vi "MdbPosEchoTableToCsv_topLevel.vi"() -> ()   [LabVIEW 2011]
uses:
  <vilib>/Utility/sysdir.llb/System Directory Type.ctl
  <vilib>/addons/database/Connection.llb/DB Tools Open Connec (String).vi
  <vilib>/addons/database/Connection.llb/DB Tools Open Connec (Path).vi
  <vilib>/addons/database/Connection.llb/Conn Get Properties.vi
  <vilib>/addons/database/_DB Variant To Data/Database Variant To Data.xnode
  <vilib>/addons/database/NI_Database_API.lvlib
panel:
  in  "Footer":string
  in  "Header":string
  in  "Database Setup":bool
  out "NumberLeft":i32 caption="Number Left To Process"
  in  "Run":bool
  in  "Shutdown":bool
  out "Number of Files":i32 caption="Number of Files to Process"
  in  "pattern":string="*.mdb" caption="File Extention Type (*.type)"
  in  "scanMDB":path caption="Database Directory to scan (non-recursive)"
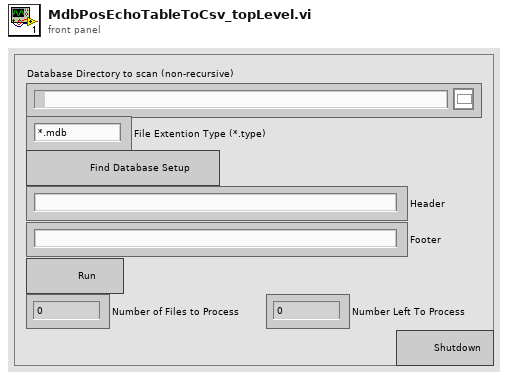
[diagram p1: front panel]
types:
  T1 = typedef "System Directory Type.ctl" = i32
  T2 = enum16{"open", "replace", "create", "open or create", "replace or create", "replace or create with confirmation"}
  T3 = typedef "NI_Database_API.lvlib/Conn ObjectReference.ctl" = refnum<k1>
  T4 = typedef "NI_Database_API.lvlib/Conn Properties.ctl" = cluster{"command timeout (s)":i32, "connection string":string, "default database":string, "provider":string}
  T5 = enum32{"invalid app kind", "Development System", "Run Time System", "Student Edition", "Embedded LabVIEW", "Evaluation", "Custom"}
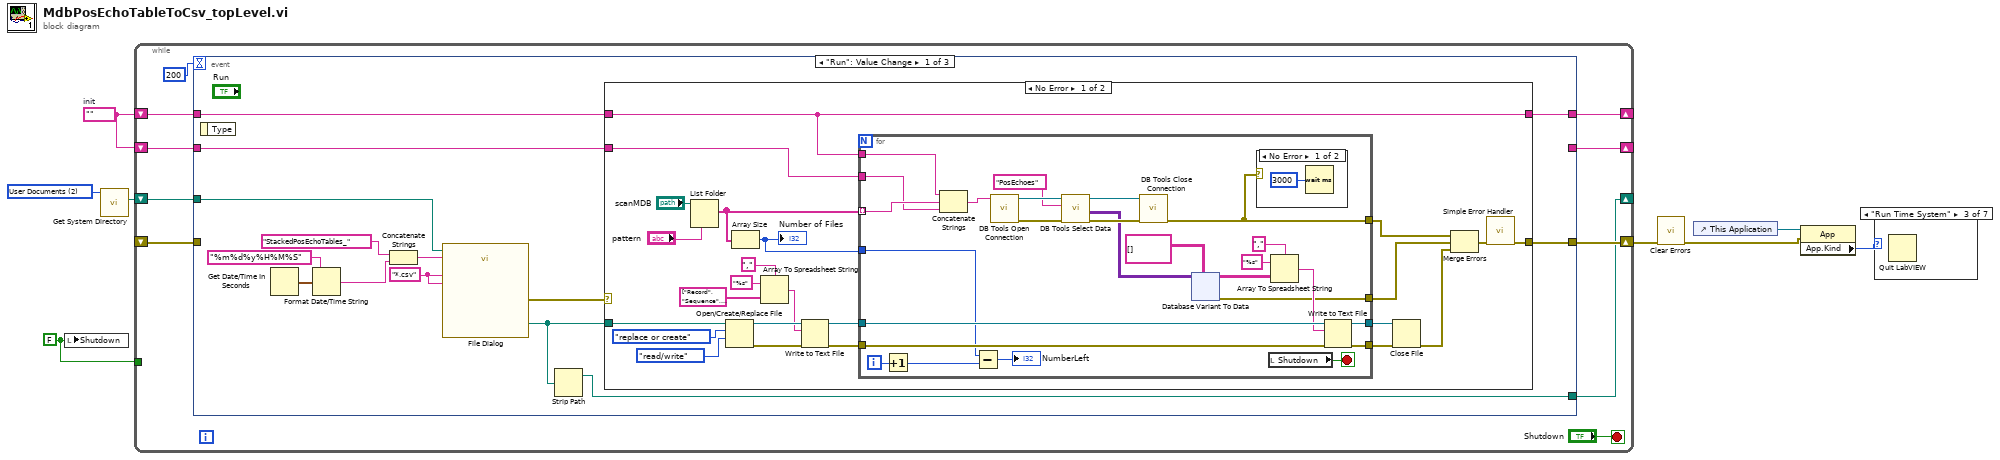
[diagram p0: block diagram]
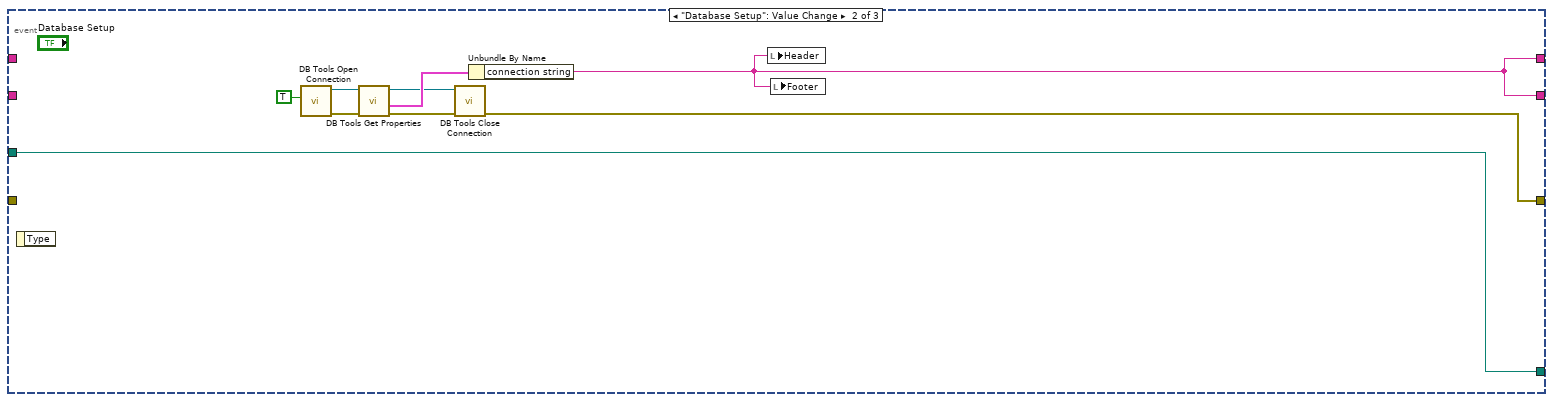
[diagram p10: hidden frame]
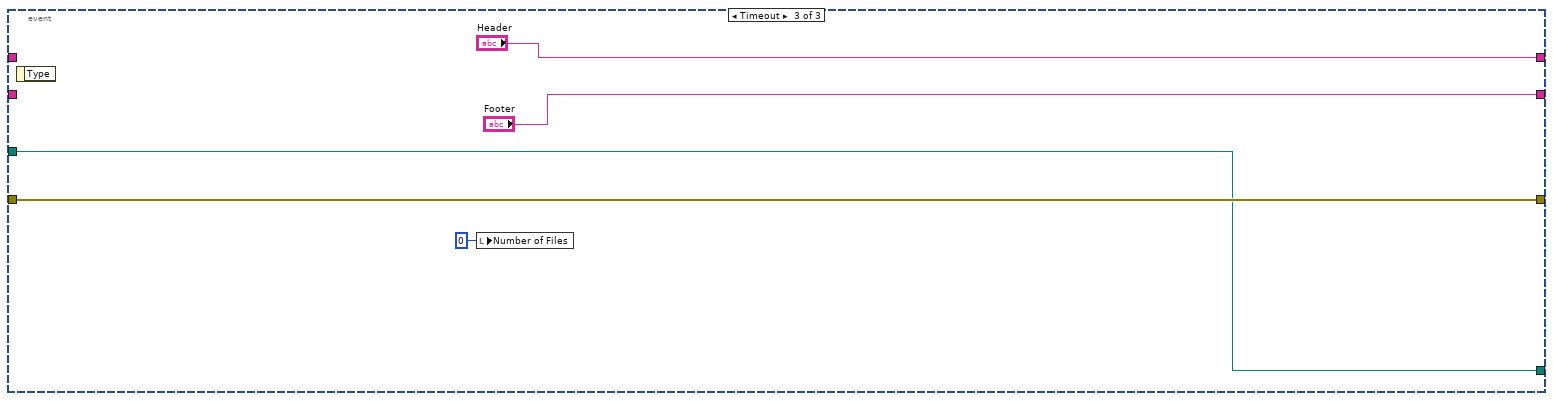
[diagram p11: hidden frame]
diagram:
  w1 = ""  # init
  w2 = FALSE ("Shutdown")
  w7 = T1 2 items=["User Home"=0, "User Desktop"=1, "User Documents"=2, "User Application Data"=3, "User Preferences"=4, "User Temporary"=5, "Public Documents"=6, "Public Application Data"=7, "Public Preferences"=8, "Public Cache"=13, "System Core Libraries"=9, "System Installed Libraries"=10, "Application Files"=11, "Boot Volume Root"=12] ("system directory type")
  n1 = local write "Shutdown"(w2) -> ()
  n2 = call <vilib>:"Get System Directory.vi"("system directory type"=w7) -> ("system directory"=w8:path)  [unwired: 10 in]
  n3 = while {
    shift-right: [w15] -> w4
    shift-left: _ -> [w14]
    shift-right: [w13] -> _
    shift-left: w1 -> [w12]
    shift-right: [w11] -> _
    shift-left: w8 -> [w18]
    tunnel: w2 -> [_]
    shift-right: [w9] -> _
    shift-left: w1 -> [w10]
    stop <- "Shutdown" stop-if-true
    n4 = event shown="[0] \"Run\": Value Change" {
      selector: _ -> [_ _ _]
      dyn-events: _ -> [_ _ _]
      timeout: 200 -> [_ _ _]
      tunnel: w18 -> [w32 w132 w142]
      tunnel: [w21 w131 w143] -> w15
      tunnel: w14 -> [_ _ w143]
      tunnel: [w25 w130 "Header"] -> w13
      tunnel: w12 -> [w23 _ _]
      tunnel: [w19 w132 w142] -> w11
      tunnel: w10 -> [w22 _ _]
      tunnel: [_ w130 "Footer"] -> w9
      event "Run": Value Change {
        w31 = "*.csv" ("pattern (all files)")
        n5 = event-data() -> ()  [unwired: 1 in, 1 out]
        n6 = Get Date/Time In Seconds() -> (seconds since 1Jan1904=w30:timestamp)
        n7 = Format Date/Time String(time format string (%c)="%m%d%y%H%M%S", seconds (now)=w30) -> (date/time string=w27:string)  [unwired: 1 in]
        n8 = Concatenate Strings("StackedPosEchoTables_" ("string"), w27) -> (w28:string)
        n9 = call "File Dialog"("start path"=w32, "default name"=w28, "pattern (all files)"=w31, "pattern label"=w31) -> ("selected path"=w20:path, "error out"=w24:errorcluster)  [unwired: 8 in, 2 out]
        n10 = Strip Path(path=w20) -> (stripped path=w19:path)  [unwired: 1 out]
        n11 = case shown="No Error" w24 {
          selector: w24 -> [_ w129]
          tunnel: w20 -> [w56 _]
          tunnel: [w34 w129] -> w21
          tunnel: w23 -> [w38 w128]
          tunnel: [w38 w128] -> w25
          tunnel: w22 -> [w35 _]
          frame No Error {
            n12 = List Folder(path="scanMDB", pattern="pattern") -> (filenames=w37:string[])  [unwired: 2 in, 3 out]
            n13 = Open/Create/Replace File(file path (use dialog)=w56, operation (0:open)=T2."replace or create", access (0:read/write)=enum16{"read/write", "read-only", "write-only"}."read/write") -> (refnum out=w51:refnum<file>, error out=w50:errorcluster)  [unwired: 3 in, 1 out]
            n14 = Array Size(array=w37) -> (size(s)=w36:i32)
            "Number of Files" <- w36
            n15 = Array To Spreadsheet String(delimiter (Tab)=",", array=string[] ["Record", "Sequence", "TransmitLoc", "Period", "SubCode", "TrackType", "EchoTime", "PosX", "PosY", "PosZ", "ElevZ", "H1Record", "H2Record", "H3Record", "H4Record", "HD1", "HD2", "HD3", "HD4"] ("Array"), 3:"%s" ("format string")) -> (spreadsheet string=w45:string)
            n16 = Write to Text File(file (use dialog)=w51, text=w45, error in=w50) -> (refnum out=w49:refnum<file>, error out=w46:errorcluster)  [unwired: 1 in, 1 out]
            n17 = for {
              tunnel: w37 -> [w59] mode=indexing
              tunnel: w49 -> [w76]
              tunnel: [w75] -> w48
              tunnel: [w74] -> w47
              tunnel: w46 -> [w73]
              tunnel: w38 -> [w67]
              tunnel: [w57] -> w42
              tunnel: [w66] -> w41
              tunnel: w36 -> [w62]
              tunnel: w35 -> [w58]
              i -> [w63]
              stop <- w64 stop-if-true
              n18 = Increment(x=w63) -> (x+1=w61:i32)
              n19 = Concatenate Strings(w67, w59, w58) -> (w82:string)
              n20 = Subtract(x=w62, y=w61) -> (x-y=→"NumberLeft":i32)
              n21 = call-poly <vilib>:"DB Tools Open Connection.vi"("connection information"=w82) -> ("error out"=w80:errorcluster, "connection reference"=w81:T3)  [unwired: 7 in]
              n22 = call <vilib>:"DB Tools Select Data.vi"("error in (no error)"=w80, "table"="PosEchoes", "connection reference"=w81) -> ("error out"=w78:errorcluster, "data"=w77:variant[][], "connection reference out"=w79:T3)  [unwired: 3 in]
              n23 = call <vilib>:"DB Tools Close Connection.vi"("error in (no error)"=w78, "connection reference"=w79) -> ("error out"=w57:errorcluster)  [unwired: 5 in]
              n24 = xnode "Database Variant To Data"("database variant"=w77, "type"=string[][] []) -> ("data"=w72:string[][], "error out"=w66:errorcluster)  [unwired: 1 in]
              n25 = case shown="No Error" w57 {
                frame No Error {
                  n26 = Wait (ms)(milliseconds to wait=u32 3000) -> ()  [unwired: 1 out]
                }
                frame Error {
                }
              }
              n27 = local read "Shutdown"() -> (w64:bool)
              n28 = Array To Spreadsheet String(delimiter (Tab)=",", array=w72, 3:"%s" ("format string")) -> (spreadsheet string=w71:string)
              n29 = Write to Text File(file (use dialog)=w76, text=w71, error in=w73) -> (refnum out=w75:refnum<file>, error out=w74:errorcluster)  [unwired: 1 in, 1 out]
            }
            n30 = Close File(refnum=w48, error in=w47) -> (error out=w40:errorcluster)  [unwired: 1 out]
            n31 = Merge Errors(w42, w41, w40) -> (w33:errorcluster)
            n32 = call <vilib>:"Simple Error Handler.vi"("error in (no error)"=w33) -> ("error out"=w34:errorcluster)  [unwired: 4 in, 4 out]
          }
          frame Error {
          }
        }
      }
      event "Database Setup": Value Change {
        n33 = event-data() -> ()  [unwired: 1 in, 1 out]
        n34 = call-poly <vilib>:"DB Tools Open Connection.vi"("prompt? (F)"=TRUE) -> ("error out"=w137:errorcluster, "connection reference"=w136:T3)  [unwired: 7 in]
        n35 = call-poly <vilib>:"DB Tools Get Properties.vi"("error in (no error)"=w137, "connection reference"=w136) -> ("error out"=w135:errorcluster, "connection properties"=w138:T4, "connection reference out"=w134:T3)  [unwired: 3 in]
        n36 = call <vilib>:"DB Tools Close Connection.vi"("error in (no error)"=w135, "connection reference"=w134) -> ("error out"=w131:errorcluster)  [unwired: 5 in]
        n37 = Unbundle By Name(w138) -> ("connection string"=w130:string)
        n38 = local write "Header"(w130) -> ()
        n39 = local write "Footer"(w130) -> ()
      }
      event Timeout {
        n40 = event-data() -> ()  [unwired: 1 in, 1 out]
        n41 = local write "Number of Files"(0 ("Number of Files")) -> ()
      }
    }
  }
  n42 = call <vilib>:"Clear Errors.vi"("error in (no error)"=w4) -> ("error out"=w3:errorcluster)  [unwired: 6 in]
  n43 = control-ref of="This Application"() -> (w6:refnum<vi>)
  n44 = property class="App"(reference=w6, error in=w3) -> ("App.Kind"=w5:T5)  [unwired: 2 out]
  n45 = case shown="\"Run Time System\"" w5 {
    frame "invalid app kind", Default {
    }
    frame "Development System" {
    }
    frame "Run Time System" {
      n46 = Quit LabVIEW() -> ()  [unwired: 1 in]
    }
    frame "Student Edition" {
    }
    frame "Embedded LabVIEW" {
    }
    frame "Evaluation" {
    }
    frame "Custom" {
    }
  }
